vi "find 2d boolean.vi"(9 "set":i32, 10 "frekans index":dbl, 11 "2D Array":dbl[][](array[numeric])) -> (3 "logical AND":bool)   [LabVIEW 2014]
panel:
  in  "pass boolean":bool[](array[boolean])
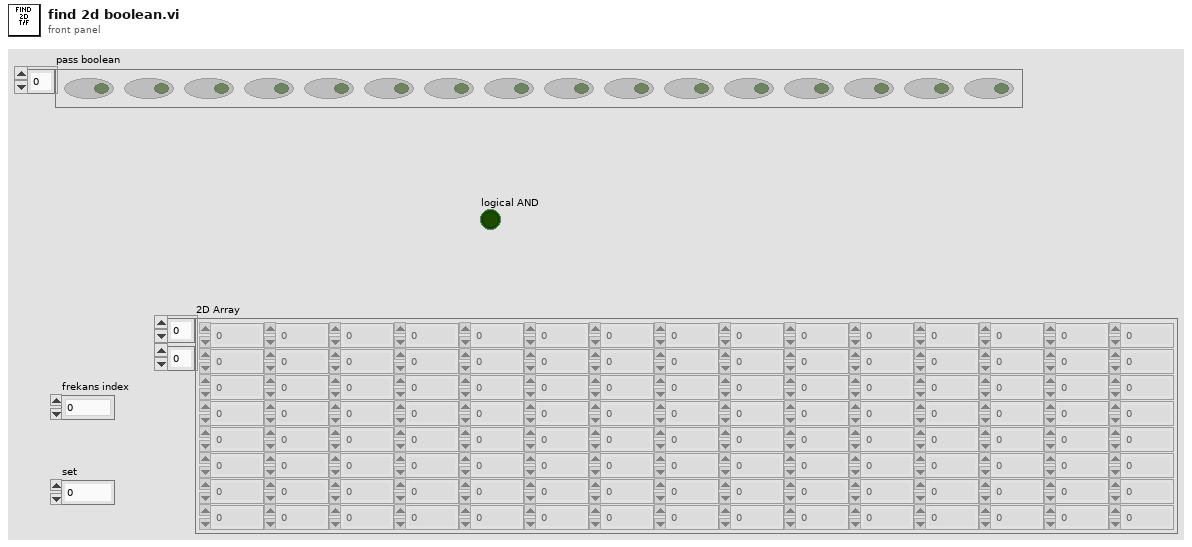
[diagram p1: front panel]
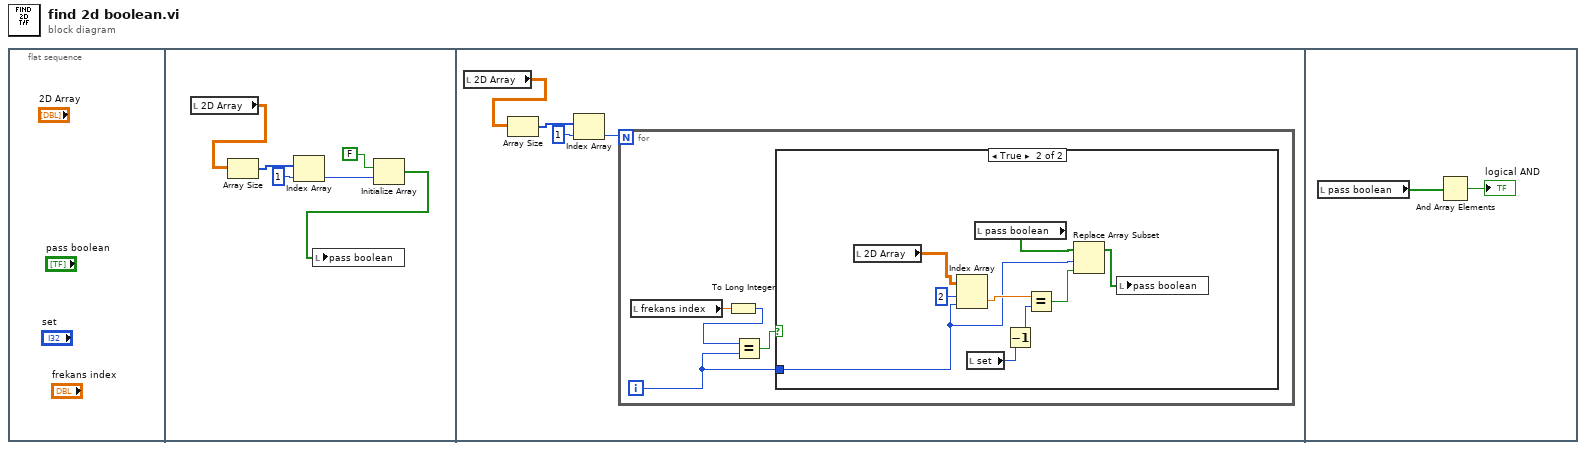
[diagram p0: block diagram]
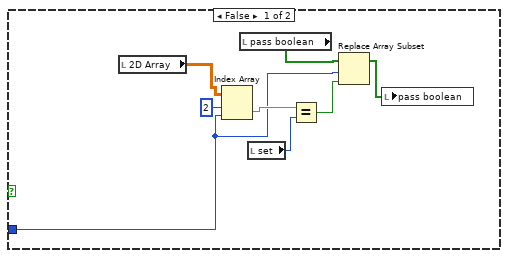
[diagram p2: hidden frame]
diagram:
  n1 = flat-sequence {
    frame #0 {
    }
    frame #1 {
      n2 = local read "2D Array"() -> (w6:dbl[][])
      n3 = Array Size(array=w6) -> (size(s)=w5:i32[])
      n4 = Index Array(array=w5, index=1) -> (element=w1:i32)
      n5 = Initialize Array(FALSE, w1) -> (w2:bool[])
      n6 = local write "pass boolean"(w2) -> ()
    }
    frame #2 {
      n7 = local read "2D Array"() -> (w10:dbl[][])
      n8 = Array Size(array=w10) -> (size(s)=w9:i32[])
      n9 = Index Array(array=w9, index=1) -> (element=w7:i32)
      n10 = for {
        N: w7 -> [_]
        i -> [w11]
        n11 = local read "frekans index"() -> (w14:dbl)
        n12 = To Long Integer(number=w14) -> (32bit integer=w13:i32)
        n13 = Equal?(x=w13, y=w11) -> (x = y?=w12:bool)
        n14 = case shown="True" w12 {
          tunnel: w11 -> [w15 w24]
          frame False {
            n15 = local read "2D Array"() -> (w22:dbl[][])
            n16 = Index Array(array=w22, index (row)=2, index (col)=w15) -> (element=w19:dbl)
            n17 = local read "pass boolean"() -> (w18:bool[])
            n18 = local read "set"() -> (w20:i32)
            n19 = Equal?(x=w19, y=w20) -> (x = y?=w17:bool)
            n20 = Replace Array Subset(array=w18, new element=w17, index=w15) -> (w16:bool[])
            n21 = local write "pass boolean"(w16) -> ()
          }
          frame True {
            n22 = local read "2D Array"() -> (w31:dbl[][])
            n23 = Index Array(array=w31, index (row)=2, index (col)=w24) -> (element=w28:dbl)
            n24 = local read "set"() -> (w29:i32)
            n25 = local read "pass boolean"() -> (w27:bool[])
            n26 = Decrement(x=w29) -> (x-1=w23:i32)
            n27 = Equal?(x=w28, y=w23) -> (x = y?=w26:bool)
            n28 = Replace Array Subset(array=w27, new element=w26, index=w24) -> (w25:bool[])
            n29 = local write "pass boolean"(w25) -> ()
          }
        }
      }
    }
    frame #3 {
      n30 = local read "pass boolean"() -> (w33:bool[])
      n31 = And Array Elements(Boolean array=w33) -> (logical AND=→"logical AND":bool)
    }
  }
